vi "DirToLocation.vi"(8 "noise":dbl format="%#_13g", 10 "Origin":T2, 11 "Position":T2) -> (3 "Direction":T1)   [LabVIEW 2017, in "Atom.lvclass"]
uses:
  Atom.lvclass
  Common/Position.ctl
  Type Defs/Direction Enum.ctl
  26161aad-ca0d-455a-a132-0b4f57b8c155.vi
  Type Defs/SB Type Defs.lvlib
  Common/Common.lvlib
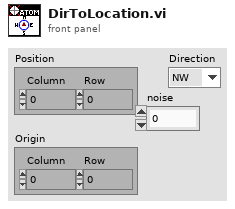
[diagram p1: front panel]
types:
  T1 = typedef "SB Type Defs.lvlib/Direction Enum.ctl" = enum16{"NW", "N", "NE", "E", "SE", "S", "SW", "W"}
  T2 = typedef "Common.lvlib/Position.ctl" = cluster{"Column":i32, "Row":i32}
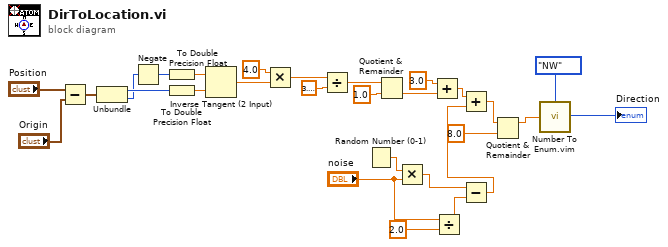
[diagram p0: block diagram]
diagram:
  n1 = Subtract(x="Position", y="Origin") -> (x-y=w26:T2)
  n2 = Unbundle(w26) -> ("Column"=w28:i32, "Row"=w27:i32)
  n3 = Negate(x=w27) -> (-x=w23:i32)
  n4 = To Double Precision Float(number=w23) -> (double precision float=w13:dbl)
  n5 = To Double Precision Float(number=w28) -> (double precision float=w14:dbl)
  n6 = Inverse Tangent (2 Input)(1:w14, 2:w13) -> (0:w19:dbl)
  n7 = Multiply(x=4.0, y=w19) -> (x*y=w18:dbl)
  n8 = Divide(x=w18, y=3.141592653589793) -> (x/y=w17:dbl)
  n9 = Random Number (0-1)() -> (number: 0 to 1=w10:dbl)
  n10 = Quotient & Remainder(x=w17, y=1.0) -> (floor(x/y)=w21:dbl)  [unwired: 1 out]
  n11 = Multiply(x=w10, y="noise") -> (x*y=w9:dbl)
  n12 = Add(x=3.0, y=w21) -> (x+y=w4:dbl)
  n13 = Divide(x="noise", y=2.0) -> (x/y=w8:dbl)
  n14 = Subtract(x=w9, y=w8) -> (x-y=w2:dbl)
  n15 = Add(x=w4, y=w2) -> (x+y=w3:dbl)
  n16 = Quotient & Remainder(x=w3, y=8.0) -> (x-y*floor(x/y)=w1:dbl)  [unwired: 1 out]
  n17 = call "Number To Enum.vim"("number"=w1, "enum type"=Direction_Enum."NW" ("Direction")) -> ("number as enum"=→"Direction":T1)
